vi "Real Inverse Matrix (Triangular).vi"(2 "matrix type":enum32{"lower triangular", "upper triangular"}(ring), 3 "A":T1) -> (0 "error":i32, 1 "Inverse Matrix":T1)   [LabVIEW 2017, in "NI_AALBase.lvlib"]
uses:
  <vilib>/Analysis/NI_AALBase.lvlib
  <vilib>/Analysis/Matrix/Datatypes/RealMatrix.ctl
  <resource>/lvanlys.dll
  <vilib>/Analysis/Matrix/NI_Matrix.lvlib
panel:
  # "Real Inverse Matrix (Triangular)"
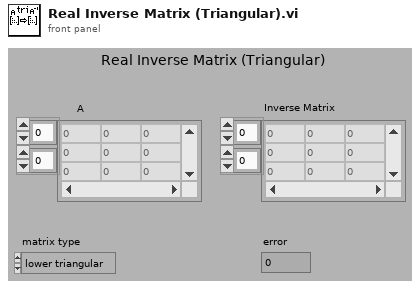
[diagram p1: front panel]
types:
  T1 = typedef "NI_Matrix.lvlib/RealMatrix.ctl" = dbl[][]
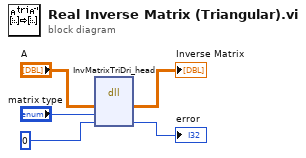
[diagram p0: block diagram]
diagram:
  n1 = dll-call lib="e:/builds/penguin/labview/branches/2017/dev/dist/resource/lvanlys.*" fn="InvMatrixTriDri_head"("A"="A", "mtype"="matrix type", 0) -> ("A"=→"Inverse Matrix":T1, →"error":i32)  [unwired: 5 in, 2 out]
